vi "New Context Menu Item.vi"(0 "NotifyIcon in":refnum<class "NotifyIcon.lvclass">, 5 "MenuItem Text":string, 9 "MenuItem Tag":string, 11 "error in (no error)":errorcluster) -> (4 "dub NotifyIcon":refnum<class "NotifyIcon.lvclass">, 8 "MenuItem":refnum<k24>, 15 "error out":errorcluster)   [LabVIEW 2016, in "NotifyIcon.lvclass"]
doc: "This VI creates a new MenuItem and assigns it the Tag from the <b>MenuItem Tag</b> input.\n\n\nStinus Olsen\nCIM Industrial Systems A/S\n22. Feb. 2011 15:05\nmailto: seo@cim.as"
uses:
  NotifyIcon.lvclass
  System.Windows.Forms
panel:
  # "This VI belongs to the NotifyIcon Toolset. \nA toolset that makes it easy to create, control and manipulate a notification icon in the notification area of the Windows taskbar.\nThe toolset requires Microsoft .NET framework 2.0\n\n\nNOTICE -- YOU MUST LEAVE THIS NOTICE IN PLACE.  PER THE TERMS OF THE LICENSE BELOW, YOU MAY SUBLICENSE THIS SOFTWARE \nIN ANY WAY THAT DOES NOT CONFLICT WITH THIS LICENSE.\n\n### BSD License (http://www.opensource.org/licenses/bsd-license.php) Begin ###\n \nCopyright (c) 2011, Stinus Olsen <seo@cim.as>\n\nAll rights reserved.\n\nRedistribution and use in source and binary forms, with or without modification, are permitted provided that the following conditions are met:\n\n    * Redistributions of source code must retain the above copyright notice, this list of conditions and the following disclaimer.\n    * Redistributions in binary form must reproduce the above copyright notice, this list of conditions and the following disclaimer in the \n       documentation and/or other materials provided with the distribution.\n    * Neither the name of CIM Industrial Systems nor the names of its contributors may be used to endorse or promote products derived \n       from this software without specific prior written permission.\n\nTHIS SOFTWARE IS PROVIDED BY THE COPYRIGHT HOLDERS AND CONTRIBUTORS \"AS IS\" AND ANY EXPRESS OR IMPLIED WARRANTIES, \nINCLUDING, BUT NOT LIMITED TO, THE IMPLIED WARRANTIES OF MERCHANTABILITY AND FITNESS FOR A PARTICULAR PURPOSE ARE \nDISCLAIMED. IN NO EVENT SHALL THE COPYRIGHT OWNER OR CONTRIBUTORS BE LIABLE FOR ANY DIRECT, INDIRECT, INCIDENTAL,\n SPECIAL, EXEMPLARY, OR CONSEQUENTIAL DAMAGES (INCLUDING, BUT NOT LIMITED TO, PROCUREMENT OF SUBSTITUTE GOODS OR \nSERVICES; LOSS OF USE, DATA, OR PROFITS; OR BUSINESS INTERRUPTION) HOWEVER CAUSED AND ON ANY THEORY OF LIABILITY, \nWHETHER IN CONTRACT, STRICT LIABILITY, OR TORT (INCLUDING NEGLIGENCE OR OTHERWISE) ARISING IN ANY WAY OUT OF THE USE \nOF THIS SOFTWARE, EVEN IF ADVISED OF THE POSSIBILITY OF SUCH DAMAGE.\n\n### BSD License End ###"
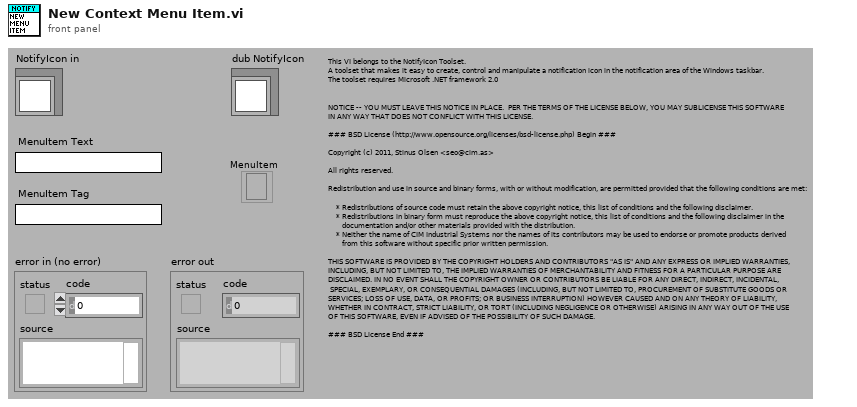
[diagram p1: front panel]
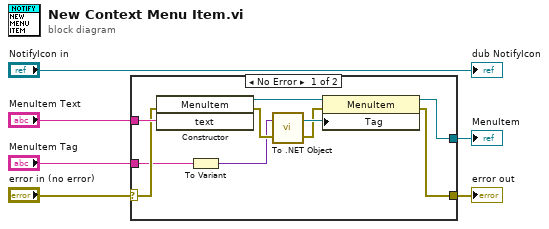
[diagram p0: block diagram]
diagram:
  n1 = case shown="No Error" "error in (no error)" {
    selector: "error in (no error)" -> [w15 w17]
    tunnel: [w7 w17] -> w5
    tunnel: "MenuItem Text" -> [w16 _]
    tunnel: [w13 _] -> w3
    tunnel: "MenuItem Tag" -> [w9 _]
    frame No Error {
      n2 = constructor class="MenuItem"(error in=w15, "text"=w16) -> (reference out=w14:refnum<k24>, error out=w11:errorcluster)  [unwired: 2 in, 2 out]
      n3 = To Variant(anything=w9) -> (Variant=w8:variant)
      n4 = call <vilib>:"To .NET Object.vi"("error in (no error)"=w11, "anything"=w8) -> ("error out"=w10:errorcluster, ".NET object"=w12:refnum<k24>)
      n5 = property class="MenuItem"(reference=w14, error in=w10, "Tag"=w12) -> (reference out=w13:refnum<k24>, error out=w7:errorcluster)
    }
    frame Error {
    }
  }
  "error out" <- w5
  "MenuItem" <- w3
  "dub NotifyIcon" <- "NotifyIcon in"
